vi "ChangeOverGui.RefNumFormatStr.vi"(0 "RefNum in":string) -> (1 "RefNum format ok?":bool, 2 "Idx":i32, 3 "RefNum out":string)   [LabVIEW 2016]
uses:
  tools/Config/Config.Global.vi
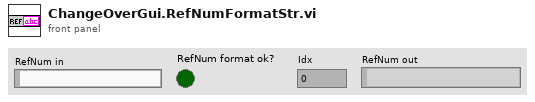
[diagram p1: front panel]
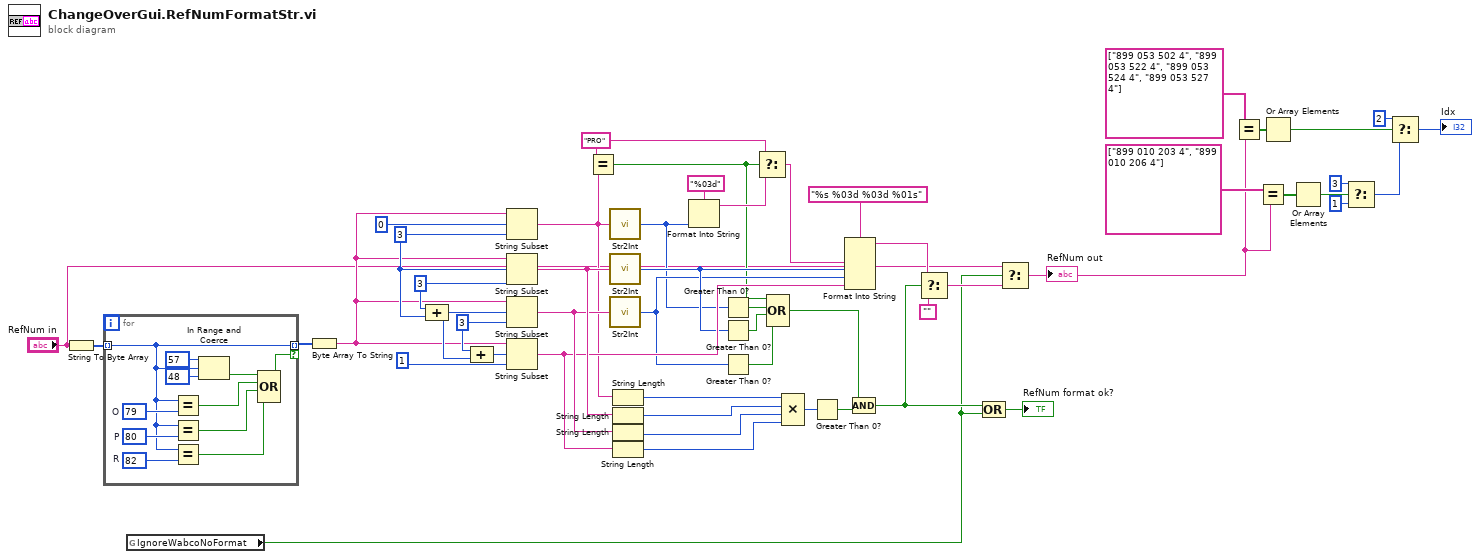
[diagram p0: block diagram]
diagram:
  w18 = "PRO" ("x")
  w47 = 3 ("length (rest)")
  w48 = 3 ("length (rest)")
  w46 = 3 ("length (rest)")
  n1 = String To Byte Array(string="RefNum in") -> (unsigned byte array=w23:u8[])
  n2 = for {
    tunnel: w23 -> [w55] mode=indexing
    tunnel: [w55] -> w22 mode=indexing if=w60
    w56 = u8 82  # R
    w57 = u8 80  # P
    w59 = u8 79  # O
    n3 = Equal?(x=w55, y=w59) -> (x = y?=w58:bool)
    n4 = Equal?(x=w55, y=w57) -> (x = y?=w54:bool)
    n5 = Equal?(x=w55, y=w56) -> (x = y?=w53:bool)
    n6 = In Range and Coerce(upper limit=u8 57, x=w55, lower limit=u8 48) -> (In Range?=w61:bool)  [unwired: 1 out]
    n7 = Compound Arithmetic op=OR(w61, w58, w54, w53) -> (w60:bool)
  }
  n8 = global read "Config.Global.vi" "IgnoreWabcoNoFormat"() -> (w2:bool)
  n9 = Byte Array To String(unsigned byte array=w22) -> (string=w21:string)
  n10 = Compound Arithmetic op=unknown(w48, w47) -> (w45:i32)
  n11 = Compound Arithmetic op=unknown(w46, w45) -> (w44:i32)
  n12 = String Subset(string=w21, offset (0)=0 ("length (rest)"), length (rest)=w47) -> (substring=w19:string)
  n13 = String Subset(string=w21, offset (0)=w47, length (rest)=w48) -> (substring=w43:string)
  n14 = String Subset(string=w21, offset (0)=w45, length (rest)=w46) -> (substring=w42:string)
  n15 = String Subset(string=w21, offset (0)=w44, length (rest)=1 ("y")) -> (substring=w20:string)
  n16 = Equal?(x=w18, y=w19) -> (x = y?=w9:bool)
  n17 = call "Str2Int.vi"("string"=w19) -> ("Numeric"=w8:i32)
  n18 = call "Str2Int.vi"("string"=w43) -> ("Numeric"=w14:i32)
  n19 = call "Str2Int.vi"("string"=w42) -> ("Numeric"=w13:i32)
  n20 = String Length(string=w19) -> (length=w41:i32)
  n21 = String Length(string=w43) -> (length=w40:i32)
  n22 = String Length(string=w42) -> (length=w39:i32)
  n23 = String Length(string=w20) -> (length=w38:i32)
  n24 = Format Into String(format string="%03d", w8) -> (resulting string=w16:string)  [unwired: 2 in, 1 out]
  n25 = Greater Than 0?(x=w8) -> (x > 0?=w12:bool)
  n26 = Greater Than 0?(x=w14) -> (x > 0?=w11:bool)
  n27 = Greater Than 0?(x=w13) -> (x > 0?=w10:bool)
  n28 = Select(t=w18, s=w9, f=w16) -> (s? t:f=w15:string)
  n29 = Compound Arithmetic op=OR(w9, w12, w11, w10) -> (w7:bool)
  n30 = Compound Arithmetic op=MULTIPLY(w41, w40, w39, w38) -> (w50:i32)
  n31 = Greater Than 0?(x=w50) -> (x > 0?=w37:bool)
  n32 = Format Into String(format string="%s %03d %03d %01s", w15, w14, w13, w20) -> (resulting string=w35:string)  [unwired: 2 in, 1 out]
  n33 = Compound Arithmetic op=AND(w7, w37) -> (w5:bool)
  n34 = Select(t=w35, s=w5, f="") -> (s? t:f=w3:string)
  n35 = Compound Arithmetic op=OR(w5, w2) -> (→"RefNum format ok?":bool)
  n36 = Select(t="RefNum in", s=w2, f=w3) -> (s? t:f=w4:string)
  "RefNum out" <- w4
  n37 = Equal?(x=string[] ["899 053 502 4", "899 053 522 4", "899 053 524 4", "899 053 527 4"], y=w4) -> (x = y?=w33:bool[])
  n38 = Equal?(x=string[] ["899 010 203 4", "899 010 206 4"], y=w4) -> (x = y?=w27:bool[])
  n39 = Or Array Elements(Boolean array=w33) -> (logical OR=w32:bool)
  n40 = Or Array Elements(Boolean array=w27) -> (logical OR=w28:bool)
  n41 = Select(t=3 ("Idx"), s=w28, f=1 ("Idx")) -> (s? t:f=w25:i32)
  n42 = Select(t=2 ("Idx"), s=w32, f=w25) -> (s? t:f=→"Idx":i32)
